vi "Ch.vi"(9 "z":u64, 10 "y":u64, 11 "x":u64) -> (3 "Ch":u64)   [LabVIEW 2020, in "NI_SHA-512.lvclass"]
doc: "Computes the SHA-2 Ch(x, y, z) function."
uses:
  <vilib>/security/Message Digest/SHA-2/SHA-512/NI_SHA-512.lvclass
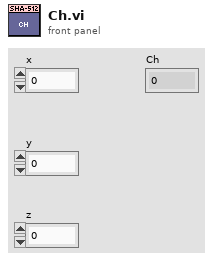
[diagram p1: front panel]
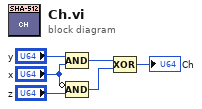
[diagram p0: block diagram]
diagram:
  n1 = Compound Arithmetic op=AND("y", "x") -> (w6:u64)
  n2 = Compound Arithmetic op=AND(invert "x", "z") -> (w5:u64)
  n3 = Compound Arithmetic op=XOR(w6, w5) -> (→"Ch":u64)
